vi "S7COMM - Evaluate Message Type.vi"(8 "error in (no error)":errorcluster, 11 "PLC Message Type":T1=3 items=["JOB"=1, "ACK"=2, "ACK_DATA"=3, "USERDATA"=7]) -> (0 "error out":errorcluster)   [LabVIEW 2014, in "S7NetCom.lvclass"]
uses:
  S7NetCom.lvclass
  S7COMM - Message Types--ring.ctl
panel:
  # "More info on https://dokuwiki.hampel-soft.com/code/hse/s7netcom\n\nCopyright (c) 2019, HAMPEL SOFTWARE ENGINEERING (HSE)\nOriginal code developed by Marc Christenson, Sisu Devices\nAll rights reserved.\n\nRedistribution and use in source and binary forms, with or without\nmodification, are permitted provided that the following conditions are met:\n\n1. Redistributions of source code must retain the above copyright\n   notice, this list of conditions and the following disclaimer.\n\n2. Redistributions in binary form must reproduce the above copyright\n   notice, this list of conditions and the following disclaimer in the\n   documentation and/or other materials provided with the distribution.\n\n3. All advertising materials mentioning features or use of this software\n   must display the following acknowledgement:\n   This product includes software developed by HAMPEL SOFTWARE ENGINEERING.\n\n4. Neither the name of HAMPEL SOFTWARE ENGINEERING nor the\n   names of its contributors may be used to endorse or promote products\n   derived from this software without specific prior written permission.\n\nTHIS SOFTWARE IS PROVIDED BY HAMPEL SOFTWARE ENGINEERING ''AS IS'' AND ANY\nEXPRESS OR IMPLIED WARRANTIES, INCLUDING, BUT NOT LIMITED TO, THE IMPLIED\nWARRANTIES OF MERCHANTABILITY AND FITNESS FOR A PARTICULAR PURPOSE ARE\nDISCLAIMED. IN NO EVENT SHALL HAMPEL SOFTWARE ENGINEERING BE LIABLE FOR ANY\nDIRECT, INDIRECT, INCIDENTAL, SPECIAL, EXEMPLARY, OR CONSEQUENTIAL DAMAGES\n(INCLUDING, BUT NOT LIMITED TO, PROCUREMENT OF SUBSTITUTE GOODS OR SERVICES;\nLOSS OF USE, DATA, OR PROFITS; OR BUSINESS INTERRUPTION) HOWEVER CAUSED AND\nON ANY THEORY OF LIABILITY, WHETHER IN CONTRACT, STRICT LIABILITY, OR TORT\n(INCLUDING NEGLIGENCE OR OTHERWISE) ARISING IN ANY WAY OUT OF THE USE OF THIS\nSOFTWARE, EVEN IF ADVISED OF THE POSSIBILITY OF SUCH DAMAGE."
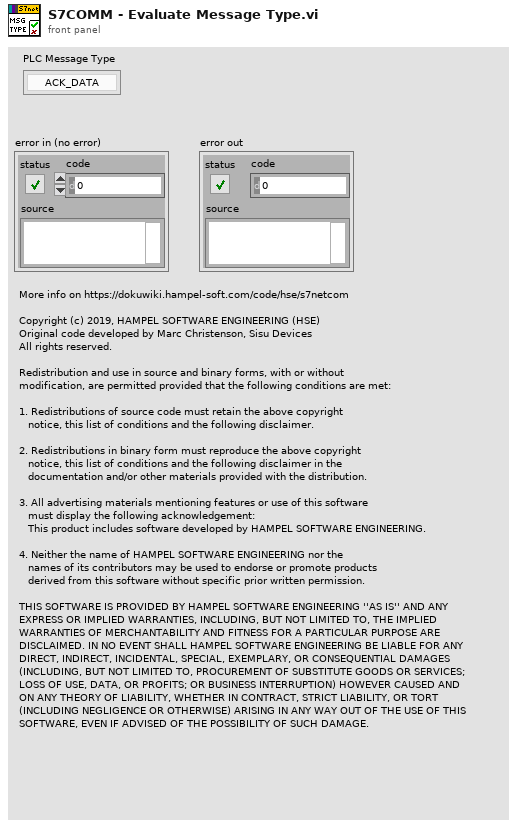
[diagram p1: front panel]
types:
  T1 = typedef "S7NetCom.lvclass/S7COMM - Message Types--ring.ctl" = u8
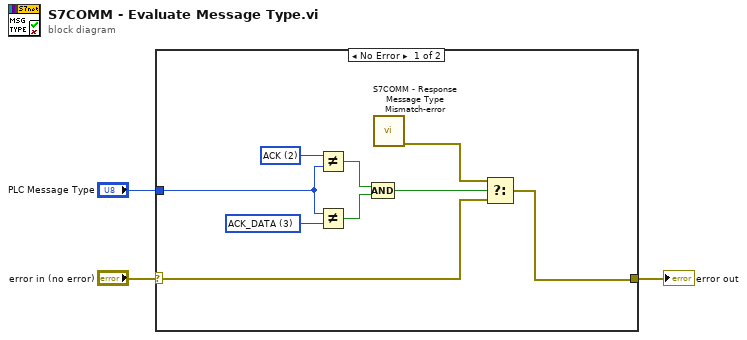
[diagram p0: block diagram]
diagram:
  n1 = case shown="No Error" "error in (no error)" {
    selector: "error in (no error)" -> [w12 w13]
    tunnel: [w11 w13] -> w3
    tunnel: "PLC Message Type" -> [w8 _]
    frame No Error {
      w6 = T1 3 items=["JOB"=1, "ACK"=2, "ACK_DATA"=3, "USERDATA"=7] ("Message Type")
      w7 = T1 2 items=["JOB"=1, "ACK"=2, "ACK_DATA"=3, "USERDATA"=7] ("Message Type")
      n2 = Not Equal?(x=w7, y=w8) -> (x != y?=w4:bool)
      n3 = Not Equal?(x=w8, y=w6) -> (x != y?=w5:bool)
      n4 = Compound Arithmetic op=AND(w4, w5) -> (w9:bool)
      n5 = call "S7COMM - Response Message Type Mismatch-error.vi"() -> ("error out"=w10:errorcluster)  [unwired: 11 in]
      n6 = Select(t=w10, s=w9, f=w12) -> (s? t:f=w11:errorcluster)
    }
    frame Error {
    }
  }
  "error out" <- w3
